vi "DisplaySpectrum.vi"() -> ()   [LabVIEW 2011]
uses:
  BeadTracker2.llb/CmdEnum_UserInterfaceCmd.ctl
  BeadTracker2.llb/GlobalVariables.vi
  <vilib>/Analysis/2dsp.llb/Real FFT.vi
  <vilib>/Analysis/NI_AALPro.lvlib
panel:
  in  "Enable?":bool
  out "Number of listeners":i32
  in  "Stop":bool
  out "FFT Z":sgl[](graph)
  out "Bead Z":sgl[](graph)
  in  "Subtract reference":bool
  in  "Reference bead#":i32
  in  "Number of frames to process":i32
  in  "Bead index":i32
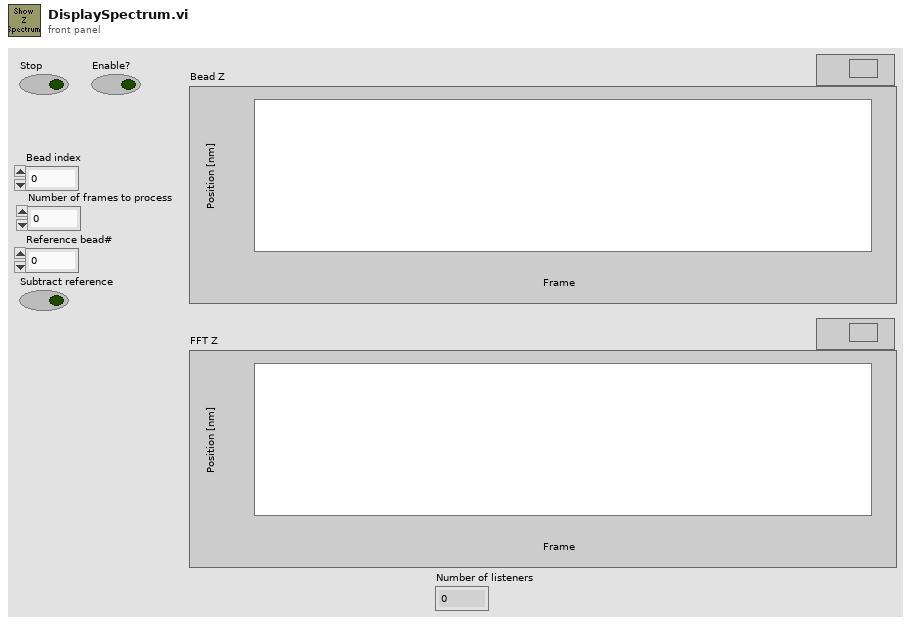
[diagram p1: front panel]
types:
  T1 = typedef "QueueListType.ctl" = cluster{"Motor In":refnum<queue>, "User Interface Image View":refnum<queue>, "Camera In":refnum<queue>, "User Interface Event Notifier":refnum<notifier>, "Initialized?":bool}
  T2 = typedef "CmdEnum_UserInterfaceCmd.ctl" = enum32{"Idle (Use for default)", "ResultTracesUpdated", "MeasureConfigUpdated", "MeasureEnd", "MeasureStart"}
  T3 = typedef "UserInterfaceEventType.ctl" = cluster{"Type":T2}
  T4 = typedef "ResultManagerInstance.ctl" = cluster{"InstancePtr":u64, "ResultManagerConfig":T5}
  T5 = typedef "ResultManagerConfig.ctl" = cluster{"Number of beads":i32, "Number of frame info columns":i32, "Result scaling":T6, "Result offset":T6, "Write Interval":i32, "Max frames in memory":i32, "Binary output (1/0)":i8}
  T6 = typedef "XYZf.ctl" = cluster{"X":sgl, "Y":sgl, "Z":sgl}
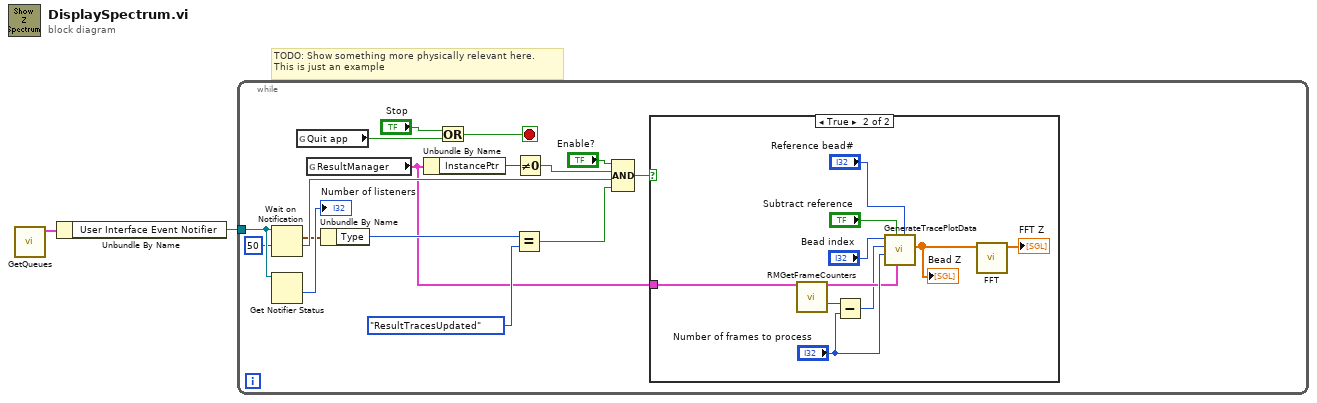
[diagram p0: block diagram]
diagram:
  # "TODO: Show something more physically relevant here.\nThis is just an example"
  n1 = call "GetQueues.vi"() -> ("Queue List"=w2:T1)  [unwired: 10 in, 1 out]
  n2 = Unbundle By Name(w2) -> ("User Interface Event Notifier"=w1:refnum<notifier>)
  n3 = while {
    tunnel: w1 -> [w9]
    stop <- w17 stop-if-true
    n4 = Wait on Notification(notifier=w9, timeout in ms (-1)=50) -> (notification=w6:T3, timed out?=w7:bool)  [unwired: 2 in, 2 out]
    n5 = Get Notifier Status(notifier=w9) -> (# waiting=→"Number of listeners":i32)  [unwired: 1 in, 4 out]
    n6 = global read "GlobalVariables.vi" "Quit app"() -> (w16:bool)
    n7 = global read "GlobalVariables.vi" "ResultManager"() -> (w4:T4)
    n8 = Unbundle By Name(w6) -> ("Type"=w5:T2)
    n9 = Unbundle By Name(w4) -> ("InstancePtr"=w14:u64)
    n10 = Or(x="Stop", y=w16) -> (x .or. y?=w17:bool)
    n11 = Equal?(x=w5, y=CmdEnum_UserInterfaceCmd."ResultTracesUpdated" ("User Interface Commands")) -> (x = y?=w11:bool)
    n12 = Not Equal To 0?(x=w14) -> (x != 0?=w12:bool)
    n13 = Compound Arithmetic op=AND("Enable?", w12, w7, w11) -> (w10:bool)
    n14 = case shown="True" w10 {
      tunnel: w4 -> [_ w19]
      frame False {
      }
      frame True {
        n15 = call "RMGetFrameCounters.vi"("ResultManager"=w19) -> ("ResultManager (out)"=w25:T4, "endFrame"=w27:i32)  [unwired: 8 in, 5 out]
        n16 = Subtract(x=w27, y="Number of frames to process") -> (x-y=w24:i32)
        n17 = call "GenerateTracePlotData.vi"("Reference bead#"="Reference bead#", "ResultManager"=w25, "Subtract reference"="Subtract reference", "Number of frames to display"="Number of frames to process", "Start frame for trace display"=w24, "Bead index"="Bead index") -> ("Bead Z"=w21:sgl[])  [unwired: 4 in, 1 out]
        "Bead Z" <- w21
        n18 = call-poly <vilib>:"FFT.vi"("X"=w21) -> ("FFT {X}"=→"FFT Z":cdb[])  [unwired: 9 in, 1 out]
      }
    }
  }
